vi "App - analyze RUS V6.vi"() -> ()   [LabVIEW 2021] (continued)
/LSCO22__130814c/5_Cooling_2nd_try/September_2014/091814/14.38000K_500_2500_2.10000V_0.00000T_Sep18-2014__05-14-56_001_091814.bin", "last mod"=timestamp(3493876496 s since 1904-01-01), "file name str"="D:\\Data\\Ultrasound\\LSCO\\LSCO22__130814c\\5_Cooling_2nd_try\\September_2014\\091814\\14.38000K_500_2500_2.10000V_0.00000T_Sep18-2014__05-14-56_001_091814.bin", "mod time(min)"=58231274.93333333, "file format"=enum."binary", "power(V)"=2.1, "Magn Field(T) "=0.0}, {"temperature"=14.384, "temperature str"="14.38400", "file path"=path "D:/Data/Ultrasound/LSCO/LSCO22__130814c/5_Cooling_2nd_try/September_2014/091814/14.38400K_500_2500_2.10000V_0.00000T_Sep18-2014__05-16-16_001_091814.bin", "last mod"=timestamp(3493876576 s since 1904-01-01), "file name str"="D:\\Data\\Ultrasound\\LSCO\\LSCO22__130814c\\5_Cooling_2nd_try\\September_2014\\091814\\14.38400K_500_2500_2.10000V_0.00000T_Sep18-2014__05-16-16_001_091814.bin", "mod time(min)"=58231276.266666666, "file format"=enum."binary", "power(V)"=2.1, "Magn Field(T) "=0.0}, {"temperature"=14.382, "temperature str"="14.38200", "file path"=path "D:/Data/Ultrasound/LSCO/LSCO22__130814c/5_Cooling_2nd_try/September_2014/091814/14.38200K_500_2500_2.10000V_0.00000T_Sep18-2014__05-17-35_001_091814.bin", "last mod"=timestamp(3493876655 s since 1904-01-01), "file name str"="D:\\Data\\Ultrasound\\LSCO\\LSCO22__130814c\\5_Cooling_2nd_try\\September_2014\\091814\\14.38200K_500_2500_2.10000V_0.00000T_Sep18-2014__05-17-35_001_091814.bin", "mod time(min)"=58231277.583333336, "file format"=enum."binary", "power(V)"=2.1, "Magn Field(T) "=0.0}, {"temperature"=14.383, "temperature str"="14.38300", "file path"=path "D:/Data/Ultrasound/LSCO/LSCO22__130814c/5_Cooling_2nd_try/September_2014/091814/14.38300K_500_2500_2.10000V_0.00000T_Sep18-2014__05-18-54_001_091814.bin", "last mod"=timestamp(3493876734 s since 1904-01-01), "file name str"="D:\\Data\\Ultrasound\\LSCO\\LSCO22__130814c\\5_Cooling_2nd_try\\September_2014\\091814\\14.38300K_500_2500_2.10000V_0.00000T_Sep18-2014__05-18-54_001_091814.bin", "mod time(min)"=58231278.9, "file format"=enum."binary", "power(V)"=2.1, "Magn Field(T) "=0.0}, {"temperature"=14.382, "temperature str"="14.38200", "file path"=path "D:/Data/Ultrasound/LSCO/LSCO22__130814c/5_Cooling_2nd_try/September_2014/091814/14.38200K_500_2500_2.10000V_0.00000T_Sep18-2014__05-20-14_001_091814.bin", "last mod"=timestamp(3493876814 s since 1904-01-01), "file name str"="D:\\Data\\Ultrasound\\LSCO\\LSCO22__130814c\\5_Cooling_2nd_try\\September_2014\\091814\\14.38200K_500_2500_2.10000V_0.00000T_Sep18-2014__05-20-14_001_091814.bin", "mod time(min)"=58231280.233333334, "file format"=enum."binary", "power(V)"=2.1, "Magn Field(T) "=0.0}, {"temperature"=14.381, "temperature str"="14.38100", "file path"=path "D:/Data/Ultrasound/LSCO/LSCO22__130814c/5_Cooling_2nd_try/September_2014/091814/14.38100K_500_2500_2.10000V_0.00000T_Sep18-2014__05-21-33_001_091814.bin", "last mod"=timestamp(3493876893 s since 1904-01-01), "file name str"="D:\\Data\\Ultrasound\\LSCO\\LSCO22__130814c\\5_Cooling_2nd_try\\September_2014\\091814\\14.38100K_500_2500_2.10000V_0.00000T_Sep18-2014__05-21-33_001_091814.bin", "mod time(min)"=58231281.55, "file format"=enum."binary", "power(V)"=2.1, "Magn Field(T) "=0.0}, {"temperature"=14.386, "temperature str"="14.38600", "file path"=path "D:/Data/Ultrasound/LSCO/LSCO22__130814c/5_Cooling_2nd_try/September_2014/091814/14.38600K_500_2500_2.10000V_0.00000T_Sep18-2014__05-22-52_001_091814.bin", "last mod"=timestamp(3493876972 s since 1904-01-01), "file name str"="D:\\Data\\Ultrasound\\LSCO\\LSCO22__130814c\\5_Cooling_2nd_try\\September_2014\\091814\\14.38600K_500_2500_2.10000V_0.00000T_Sep18-2014__05-22-52_001_091814.bin", "mod time(min)"=58231282.86666667, "file format"=enum."binary", "power(V)"=2.1, "Magn Field(T) "=0.0}, {"temperature"=14.389, "temperature str"="14.38900", "file path"=path "D:/Data/Ultrasound/LSCO/LSCO22__130814c/5_Cooling_2nd_try/September_2014/091814/14.38900K_500_2500_2.10000V_0.00000T_Sep18-2014__05-24-12_001_091814.bin", "last mod"=timestamp(3493877052 s since 1904-01-01), "file name str"="D:\\Data\\Ultrasound\\LSCO\\LSCO22__130814c\\5_Cooling_2nd_try\\September_2014\\091814\\14.38900K_500_2500_2.10000V_0.00000T_Sep18-2014__05-24-12_001_091814.bin", "mod time(min)"=58231284.2, "file format"=enum."binary", "power(V)"=2.1, "Magn Field(T) "=0.0}, {"temperature"=14.392, "temperature str"="14.39200", "file path"=path "D:/Data/Ultrasound/LSCO/LSCO22__130814c/5_Cooling_2nd_try/September_2014/091814/14.39200K_500_2500_2.10000V_0.00000T_Sep18-2014__05-25-31_001_091814.bin", "last mod"=timestamp(3493877131 s since 1904-01-01), "file name str"="D:\\Data\\Ultrasound\\LSCO\\LSCO22__130814c\\5_Cooling_2nd_try\\September_2014\\091814\\14.39200K_500_2500_2.10000V_0.00000T_Sep18-2014__05-25-31_001_091814.bin", "mod time(min)"=58231285.516666666, "file format"=enum."binary", "power(V)"=2.1, "Magn Field(T) "=0.0}, {"temperature"=14.395, "temperature str"="14.39500", "file path"=path "D:/Data/Ultrasound/LSCO/LSCO22__130814c/5_Cooling_2nd_try/September_2014/091814/14.39500K_500_2500_2.10000V_0.00000T_Sep18-2014__05-26-51_001_091814.bin", "last mod"=timestamp(3493877211 s since 1904-01-01), "file name str"="D:\\Data\\Ultrasound\\LSCO\\LSCO22__130814c\\5_Cooling_2nd_try\\September_2014\\091814\\14.39500K_500_2500_2.10000V_0.00000T_Sep18-2014__05-26-51_001_091814.bin", "mod time(min)"=58231286.85, "file format"=enum."binary", "power(V)"=2.1, "Magn Field(T) "=0.0}, {"temperature"=14.397, "temperature str"="14.39700", "file path"=path "D:/Data/Ultrasound/LSCO/LSCO22__130814c/5_Cooling_2nd_try/September_2014/091814/14.39700K_500_2500_2.10000V_0.00000T_Sep18-2014__05-28-10_001_091814.bin", "last mod"=timestamp(3493877290 s since 1904-01-01), "file name str"="D:\\Data\\Ultrasound\\LSCO\\LSCO22__130814c\\5_Cooling_2nd_try\\September_2014\\091814\\14.39700K_500_2500_2.10000V_0.00000T_Sep18-2014__05-28-10_001_091814.bin", "mod time(min)"=58231288.166666664, "file format"=enum."binary", "power(V)"=2.1, "Magn Field(T) "=0.0}, {"temperature"=14.399, "temperature str"="14.39900", "file path"=path "D:/Data/Ultrasound/LSCO/LSCO22__130814c/5_Cooling_2nd_try/September_2014/091814/14.39900K_500_2500_2.10000V_0.00000T_Sep18-2014__05-29-29_001_091814.bin", "last mod"=timestamp(3493877369 s since 1904-01-01), "file name str"="D:\\Data\\Ultrasound\\LSCO\\LSCO22__130814c\\5_Cooling_2nd_try\\September_2014\\091814\\14.39900K_500_2500_2.10000V_0.00000T_Sep18-2014__05-29-29_001_091814.bin", "mod time(min)"=58231289.483333334, "file format"=enum."binary", "power(V)"=2.1, "Magn Field(T) "=0.0}, {"temperature"=14.4, "temperature str"="14.40000", "file path"=path "D:/Data/Ultrasound/LSCO/LSCO22__130814c/5_Cooling_2nd_try/September_2014/091814/14.40000K_500_2500_2.10000V_0.00000T_Sep18-2014__05-30-49_001_091814.bin", "last mod"=timestamp(3493877449 s since 1904-01-01), "file name str"="D:\\Data\\Ultrasound\\LSCO\\LSCO22__130814c\\5_Cooling_2nd_try\\September_2014\\091814\\14.40000K_500_2500_2.10000V_0.00000T_Sep18-2014__05-30-49_001_091814.bin", "mod time(min)"=58231290.81666667, "file format"=enum."binary", "power(V)"=2.1, "Magn Field(T) "=0.0}, {"temperature"=14.404, "temperature str"="14.40400", "file path"=path "D:/Data/Ultrasound/LSCO/LSCO22__130814c/5_Cooling_2nd_try/September_2014/091814/14.40400K_500_2500_2.10000V_0.00000T_Sep18-2014__05-32-08_001_091814.bin", "last mod"=timestamp(3493877528 s since 1904-01-01), "file name str"="D:\\Data\\Ultrasound\\LSCO\\LSCO22__130814c\\5_Cooling_2nd_try\\September_2014\\091814\\14.40400K_500_2500_2.10000V_0.00000T_Sep18-2014__05-32-08_001_091814.bin", "mod time(min)"=58231292.13333333, "file format"=enum."binary", "power(V)"=2.1, "Magn Field(T) "=0.0}, {"temperature"=14.405, "temperature str"="14.40500", "file path"=path "D:/Data/Ultrasound/LSCO/LSCO22__130814c/5_Cooling_2nd_try/September_2014/091814/14.40500K_500_2500_2.10000V_0.00000T_Sep18-2014__05-33-28_001_091814.bin", "last mod"=timestamp(3493877608 s since 1904-01-01), "file name str"="D:\\Data\\Ultrasound\\LSCO\\LSCO22__130814c\\5_Cooling_2nd_try\\September_2014\\091814\\14.40500K_500_2500_2.10000V_0.00000T_Sep18-2014__05-33-28_001_091814.bin", "mod time(min)"=58231293.46666667, "file format"=enum."binary", "power(V)"=2.1, "Magn Field(T) "=0.0}, {"temperature"=14.407, "temperature str"="14.40700", "file path"=path "D:/Data/Ultrasound/LSCO/LSCO22__130814c/5_Cooling_2nd_try/September_2014/091814/14.40700K_500_2500_2.10000V_0.00000T_Sep18-2014__05-34-47_001_091814.bin", "last mod"=timestamp(3493877687 s since 1904-01-01), "file name str"="D:\\Data\\Ultrasound\\LSCO\\LSCO22__130814c\\5_Cooling_2nd_try\\September_2014\\091814\\14.40700K_500_2500_2.10000V_0.00000T_Sep18-2014__05-34-47_001_091814.bin", "mod time(min)"=58231294.78333333, "file format"=enum."binary", "power(V)"=2.1, "Magn Field(T) "=0.0}, {"temperature"=14.411, "temperature str"="14.41100", "file path"=path "D:/Data/Ultrasound/LSCO/LSCO22__130814c/5_Cooling_2nd_try/September_2014/091814/14.41100K_500_2500_2.10000V_0.00000T_Sep18-2014__05-36-06_001_091814.bin", "last mod"=timestamp(3493877766 s since 1904-01-01), "file name str"="D:\\Data\\Ultrasound\\LSCO\\LSCO22__130814c\\5_Cooling_2nd_try\\September_2014\\091814\\14.41100K_500_2500_2.10000V_0.00000T_Sep18-2014__05-36-06_001_091814.bin", "mod time(min)"=58231296.1, "file format"=enum."binary", "power(V)"=2.1, "Magn Field(T) "=0.0}, {"temperature"=14.416, "temperature str"="14.41600", "file path"=path "D:/Data/Ultrasound/LSCO/LSCO22__130814c/5_Cooling_2nd_try/September_2014/091814/14.41600K_500_2500_2.10000V_0.00000T_Sep18-2014__05-37-26_001_091814.bin", "last mod"=timestamp(3493877846 s since 1904-01-01), "file name str"="D:\\Data\\Ultrasound\\LSCO\\LSCO22__130814c\\5_Cooling_2nd_try\\September_2014\\091814\\14.41600K_500_2500_2.10000V_0.00000T_Sep18-2014__05-37-26_001_091814.bin", "mod time(min)"=58231297.43333333, "file format"=enum."binary", "power(V)"=2.1, "Magn Field(T) "=0.0}, {"temperature"=14.42, "temperature str"="14.42000", "file path"=path "D:/Data/Ultrasound/LSCO/LSCO22__130814c/5_Cooling_2nd_try/September_2014/091814/14.42000K_500_2500_2.10000V_0.00000T_Sep18-2014__05-38-45_001_091814.bin", "last mod"=timestamp(3493877925 s since 1904-01-01), "file name str"="D:\\Data\\Ultrasound\\LSCO\\LSCO22__130814c\\5_Cooling_2nd_try\\September_2014\\091814\\14.42000K_500_2500_2.10000V_0.00000T_Sep18-2014__05-38-45_001_091814.bin", "mod time(min)"=58231298.75, "file format"=enum."binary", "power(V)"=2.1, "Magn Field(T) "=0.0}, {"temperature"=14.42, "temperature str"="14.42000", "file path"=path "D:/Data/Ultrasound/LSCO/LSCO22__130814c/5_Cooling_2nd_try/September_2014/091814/14.42000K_500_2500_2.10000V_0.00000T_Sep18-2014__05-40-04_001_091814.bin", "last mod"=timestamp(3493878004 s since 1904-01-01), "file name str"="D:\\Data\\Ultrasound\\LSCO\\LSCO22__130814c\\5_Cooling_2nd_try\\September_2014\\091814\\14.42000K_500_2500_2.10000V_0.00000T_Sep18-2014__05-40-04_001_091814.bin", "mod time(min)"=58231300.06666667, "file format"=enum."binary", "power(V)"=2.1, "Magn Field(T) "=0.0}, {"temperature"=14.42, "temperature str"="14.42000", "file path"=path "D:/Data/Ultrasound/LSCO/LSCO22__130814c/5_Cooling_2nd_try/September_2014/091814/14.42000K_500_2500_2.10000V_0.00000T_Sep18-2014__05-41-24_001_091814.bin", "last mod"=timestamp(3493878084 s since 1904-01-01), "file name str"="D:\\Data\\Ultrasound\\LSCO\\LSCO22__130814c\\5_Cooling_2nd_try\\September_2014\\091814\\14.42000K_500_2500_2.10000V_0.00000T_Sep18-2014__05-41-24_001_091814.bin", "mod time(min)"=58231301.4, "file format"=enum."binary", "power(V)"=2.1, "Magn Field(T) "=0.0}, {"temperature"=14.42, "temperature str"="14.42000", "file path"=path "D:/Data/Ultrasound/LSCO/LSCO22__130814c/5_Cooling_2nd_try/September_2014/091814/14.42000K_500_2500_2.10000V_0.00000T_Sep18-2014__05-42-43_001_091814.bin", "last mod"=timestamp(3493878163 s since 1904-01-01), "file name str"="D:\\Data\\Ultrasound\\LSCO\\LSCO22__130814c\\5_Cooling_2nd_try\\September_2014\\091814\\14.42000K_500_2500_2.10000V_0.00000T_Sep18-2014__05-42-43_001_091814.bin", "mod time(min)"=58231302.71666667, "file format"=enum."binary", "power(V)"=2.1, "Magn Field(T) "=0.0}, {"temperature"=14.426, "temperature str"="14.42600", "file path"=path "D:/Data/Ultrasound/LSCO/LSCO22__130814c/5_Cooling_2nd_try/September_2014/091814/14.42600K_500_2500_2.10000V_0.00000T_Sep18-2014__05-44-03_001_091814.bin", "last mod"=timestamp(3493878243 s since 1904-01-01), "file name str"="D:\\Data\\Ultrasound\\LSCO\\LSCO22__130814c\\5_Cooling_2nd_try\\September_2014\\091814\\14.42600K_500_2500_2.10000V_0.00000T_Sep18-2014__05-44-03_001_091814.bin", "mod time(min)"=58231304.05, "file format"=enum."binary", "power(V)"=2.1, "Magn Field(T) "=0.0}, {"temperature"=14.427, "temperature str"="14.42700", "file path"=path "D:/Data/Ultrasound/LSCO/LSCO22__130814c/5_Cooling_2nd_try/September_2014/091814/14.42700K_500_2500_2.10000V_0.00000T_Sep18-2014__05-45-22_001_091814.bin", "last mod"=timestamp(3493878322 s since 1904-01-01), "file name str"="D:\\Data\\Ultrasound\\LSCO\\LSCO22__130814c\\5_Cooling_2nd_try\\September_2014\\091814\\14.42700K_500_2500_2.10000V_0.00000T_Sep18-2014__05-45-22_001_091814.bin", "mod time(min)"=58231305.36666667, "file format"=enum."binary", "power(V)"=2.1, "Magn Field(T) "=0.0}, {"temperature"=14.431, "temperature str"="14.43100", "file path"=path "D:/Data/Ultrasound/LSCO/LSCO22__130814c/5_Cooling_2nd_try/September_2014/091814/14.43100K_500_2500_2.10000V_0.00000T_Sep18-2014__05-46-41_001_091814.bin", "last mod"=timestamp(3493878401 s since 1904-01-01), "file name str"="D:\\Data\\Ultrasound\\LSCO\\LSCO22__130814c\\5_Cooling_2nd_try\\September_2014\\091814\\14.43100K_500_2500_2.10000V_0.00000T_Sep18-2014__05-46-41_001_091814.bin", "mod time(min)"=58231306.68333333, "file format"=enum."binary", "power(V)"=2.1, "Magn Field(T) "=0.0}, {"temperature"=14.43, "temperature str"="14.43000", "file path"=path "D:/Data/Ultrasound/LSCO/LSCO22__130814c/5_Cooling_2nd_try/September_2014/091814/14.43000K_500_2500_2.10000V_0.00000T_Sep18-2014__05-48-01_001_091814.bin", "last mod"=timestamp(3493878481 s since 1904-01-01), "file name str"="D:\\Data\\Ultrasound\\LSCO\\LSCO22__130814c\\5_Cooling_2nd_try\\September_2014\\091814\\14.43000K_500_2500_2.10000V_0.00000T_Sep18-2014__05-48-01_001_091814.bin", "mod time(min)"=58231308.016666666, "file format"=enum."binary", "power(V)"=2.1, "Magn Field(T) "=0.0}, {"temperature"=14.431, "temperature str"="14.43100", "file path"=path "D:/Data/Ultrasound/LSCO/LSCO22__130814c/5_Cooling_2nd_try/September_2014/091814/14.43100K_500_2500_2.10000V_0.00000T_Sep18-2014__05-49-20_001_091814.bin", "last mod"=timestamp(3493878560 s since 1904-01-01), "file name str"="D:\\Data\\Ultrasound\\LSCO\\LSCO22__130814c\\5_Cooling_2nd_try\\September_2014\\091814\\14.43100K_500_2500_2.10000V_0.00000T_Sep18-2014__05-49-20_001_091814.bin", "mod time(min)"=58231309.333333336, "file format"=enum."binary", "power(V)"=2.1, "Magn Field(T) "=0.0}, {"temperature"=14.433, "temperature str"="14.43300", "file path"=path "D:/Data/Ultrasound/LSCO/LSCO22__130814c/5_Cooling_2nd_try/September_2014/091814/14.43300K_500_2500_2.10000V_0.00000T_Sep18-2014__05-50-40_001_091814.bin", "last mod"=timestamp(3493878640 s since 1904-01-01), "file name str"="D:\\Data\\Ultrasound\\LSCO\\LSCO22__130814c\\5_Cooling_2nd_try\\September_2014\\091814\\14.43300K_500_2500_2.10000V_0.00000T_Sep18-2014__05-50-40_001_091814.bin", "mod time(min)"=58231310.666666664, "file format"=enum."binary", "power(V)"=2.1, "Magn Field(T) "=0.0}, {"temperature"=14.438, "temperature str"="14.43800", "file path"=path "D:/Data/Ultrasound/LSCO/LSCO22__130814c/5_Cooling_2nd_try/September_2014/091814/14.43800K_500_2500_2.10000V_0.00000T_Sep18-2014__05-51-59_001_091814.bin", "last mod"=timestamp(3493878719 s since 1904-01-01), "file name str"="D:\\Data\\Ultrasound\\LSCO\\LSCO22__130814c\\5_Cooling_2nd_try\\September_2014\\091814\\14.43800K_500_2500_2.10000V_0.00000T_Sep18-2014__05-51-59_001_091814.bin", "mod time(min)"=58231311.983333334, "file format"=enum."binary", "power(V)"=2.1, "Magn Field(T) "=0.0}, {"temperature"=14.434, "temperature str"="14.43400", "file path"=path "D:/Data/Ultrasound/LSCO/LSCO22__130814c/5_Cooling_2nd_try/September_2014/091814/14.43400K_500_2500_2.10000V_0.00000T_Sep18-2014__05-53-18_001_091814.bin", "last mod"=timestamp(3493878798 s since 1904-01-01), "file name str"="D:\\Data\\Ultrasound\\LSCO\\LSCO22__130814c\\5_Cooling_2nd_try\\September_2014\\091814\\14.43400K_500_2500_2.10000V_0.00000T_Sep18-2014__05-53-18_001_091814.bin", "mod time(min)"=58231313.3, "file format"=enum."binary", "power(V)"=2.1, "Magn Field(T) "=0.0}, {"temperature"=14.438, "temperature str"="14.43800", "file path"=path "D:/Data/Ultrasound/LSCO/LSCO22__130814c/5_Cooling_2nd_try/September_2014/091814/14.43800K_500_2500_2.10000V_0.00000T_Sep18-2014__05-54-38_001_091814.bin", "last mod"=timestamp(3493878878 s since 1904-01-01), "file name str"="D:\\Data\\Ultrasound\\LSCO\\LSCO22__130814c\\5_Cooling_2nd_try\\September_2014\\091814\\14.43800K_500_2500_2.10000V_0.00000T_Sep18-2014__05-54-38_001_091814.bin", "mod time(min)"=58231314.63333333, "file format"=enum."binary", "power(V)"=2.1, "Magn Field(T) "=0.0}, {"temperature"=14.441, "temperature str"="14.44100", "file path"=path "D:/Data/Ultrasound/LSCO/LSCO22__130814c/5_Cooling_2nd_try/September_2014/091814/14.44100K_500_2500_2.10000V_0.00000T_Sep18-2014__05-55-57_001_091814.bin", "last mod"=timestamp(3493878957 s since 1904-01-01), "file name str"="D:\\Data\\Ultrasound\\LSCO\\LSCO22__130814c\\5_Cooling_2nd_try\\September_2014\\091814\\14.44100K_500_2500_2.10000V_0.00000T_Sep18-2014__05-55-57_001_091814.bin", "mod time(min)"=58231315.95, "file format"=enum."binary", "power(V)"=2.1, "Magn Field(T) "=0.0}, {"temperature"=14.441, "temperature str"="14.44100", "file path"=path "D:/Data/Ultrasound/LSCO/LSCO22__130814c/5_Cooling_2nd_try/September_2014/091814/14.44100K_500_2500_2.10000V_0.00000T_Sep18-2014__05-57-16_001_091814.bin", "last mod"=timestamp(3493879036 s since 1904-01-01), "file name str"="D:\\Data\\Ultrasound\\LSCO\\LSCO22__130814c\\5_Cooling_2nd_try\\September_2014\\091814\\14.44100K_500_2500_2.10000V_0.00000T_Sep18-2014__05-57-16_001_091814.bin", "mod time(min)"=58231317.266666666, "file format"=enum."binary", "power(V)"=2.1, "Magn Field(T) "=0.0}, {"temperature"=14.444, "temperature str"="14.44400", "file path"=path "D:/Data/Ultrasound/LSCO/LSCO22__130814c/5_Cooling_2nd_try/September_2014/091814/14.44400K_500_2500_2.10000V_0.00000T_Sep18-2014__05-58-36_001_091814.bin", "last mod"=timestamp(3493879116 s since 1904-01-01), "file name str"="D:\\Data\\Ultrasound\\LSCO\\LSCO22__130814c\\5_Cooling_2nd_try\\September_2014\\091814\\14.44400K_500_2500_2.10000V_0.00000T_Sep18-2014__05-58-36_001_091814.bin", "mod time(min)"=58231318.6, "file format"=enum."binary", "power(V)"=2.1, "Magn Field(T) "=0.0}, {"temperature"=14.44, "temperature str"="14.44000", "file path"=path "D:/Data/Ultrasound/LSCO/LSCO22__130814c/5_Cooling_2nd_try/September_2014/091814/14.44000K_500_2500_2.10000V_0.00000T_Sep18-2014__05-59-55_001_091814.bin", "last mod"=timestamp(3493879195 s since 1904-01-01), "file name str"="D:\\Data\\Ultrasound\\LSCO\\LSCO22__130814c\\5_Cooling_2nd_try\\September_2014\\091814\\14.44000K_500_2500_2.10000V_0.00000T_Sep18-2014__05-59-55_001_091814.bin", "mod time(min)"=58231319.916666664, "file format"=enum."binary", "power(V)"=2.1, "Magn Field(T) "=0.0}, {"temperature"=14.446, "temperature str"="14.44600", "file path"=path "D:/Data/Ultrasound/LSCO/LSCO22__130814c/5_Cooling_2nd_try/September_2014/091814/14.44600K_500_2500_2.10000V_0.00000T_Sep18-2014__06-01-15_001_091814.bin", "last mod"=timestamp(3493879275 s since 1904-01-01), "file name str"="D:\\Data\\Ultrasound\\LSCO\\LSCO22__130814c\\5_Cooling_2nd_try\\September_2014\\091814\\14.44600K_500_2500_2.10000V_0.00000T_Sep18-2014__06-01-15_001_091814.bin", "mod time(min)"=58231321.25, "file format"=enum."binary", "power(V)"=2.1, "Magn Field(T) "=0.0}, {"temperature"=14.449, "temperature str"="14.44900", "file path"=path "D:/Data/Ultrasound/LSCO/LSCO22__130814c/5_Cooling_2nd_try/September_2014/091814/14.44900K_500_2500_2.10000V_0.00000T_Sep18-2014__06-02-34_001_091814.bin", "last mod"=timestamp(3493879354 s since 1904-01-01), "file name str"="D:\\Data\\Ultrasound\\LSCO\\LSCO22__130814c\\5_Cooling_2nd_try\\September_2014\\091814\\14.44900K_500_2500_2.10000V_0.00000T_Sep18-2014__06-02-34_001_091814.bin", "mod time(min)"=58231322.56666667, "file format"=enum."binary", "power(V)"=2.1, "Magn Field(T) "=0.0}, {"temperature"=14.447, "temperature str"="14.44700", "file path"=path "D:/Data/Ultrasound/LSCO/LSCO22__130814c/5_Cooling_2nd_try/September_2014/091814/14.44700K_500_2500_2.10000V_0.00000T_Sep18-2014__06-03-53_001_091814.bin", "last mod"=timestamp(3493879433 s since 1904-01-01), "file name str"="D:\\Data\\Ultrasound\\LSCO\\LSCO22__130814c\\5_Cooling_2nd_try\\September_2014\\091814\\14.44700K_500_2500_2.10000V_0.00000T_Sep18-2014__06-03-53_001_091814.bin", "mod time(min)"=58231323.88333333, "file format"=enum."binary", "power(V)"=2.1, "Magn Field(T) "=0.0}, {"temperature"=14.448, "temperature str"="14.44800", "file path"=path "D:/Data/Ultrasound/LSCO/LSCO22__130814c/5_Cooling_2nd_try/September_2014/091814/14.44800K_500_2500_2.10000V_0.00000T_Sep18-2014__06-05-13_001_091814.bin", "last mod"=timestamp(3493879513 s since 1904-01-01), "file name str"="D:\\Data\\Ultrasound\\LSCO\\LSCO22__130814c\\5_Cooling_2nd_try\\September_2014\\091814\\14.44800K_500_2500_2.10000V_0.00000T_Sep18-2014__06-05-13_001_091814.bin", "mod time(min)"=58231325.21666667, "file format"=enum."binary", "power(V)"=2.1, "Magn Field(T) "=0.0}, {"temperature"=14.453, "temperature str"="14.45300", "file path"=path "D:/Data/Ultrasound/LSCO/LSCO22__130814c/5_Cooling_2nd_try/September_2014/091814/14.45300K_500_2500_2.10000V_0.00000T_Sep18-2014__06-06-32_001_091814.bin", "last mod"=timestamp(3493879592 s since 1904-01-01), "file name str"="D:\\Data\\Ultrasound\\LSCO\\LSCO22__130814c\\5_Cooling_2nd_try\\September_2014\\091814\\14.45300K_500_2500_2.10000V_0.00000T_Sep18-2014__06-06-32_001_091814.bin", "mod time(min)"=58231326.53333333, "file format"=enum."binary", "power(V)"=2.1, "Magn Field(T) "=0.0}, {"temperature"=14.45, "temperature str"="14.45000", "file path"=path "D:/Data/Ultrasound/LSCO/LSCO22__130814c/5_Cooling_2nd_try/September_2014/091814/14.45000K_500_2500_2.10000V_0.00000T_Sep18-2014__06-07-51_001_091814.bin", "last mod"=timestamp(3493879671 s since 1904-01-01), "file name str"="D:\\Data\\Ultrasound\\LSCO\\LSCO22__130814c\\5_Cooling_2nd_try\\September_2014\\091814\\14.45000K_500_2500_2.10000V_0.00000T_Sep18-2014__06-07-51_001_091814.bin", "mod time(min)"=58231327.85, "file format"=enum."binary", "power(V)"=2.1, "Magn Field(T) "=0.0}, {"temperature"=14.451, "temperature str"="14.45100", "file path"=path "D:/Data/Ultrasound/LSCO/LSCO22__130814c/5_Cooling_2nd_try/September_2014/091814/14.45100K_500_2500_2.10000V_0.00000T_Sep18-2014__06-09-11_001_091814.bin", "last mod"=timestamp(3493879751 s since 1904-01-01), "file name str"="D:\\Data\\Ultrasound\\LSCO\\LSCO22__130814c\\5_Cooling_2nd_try\\September_2014\\091814\\14.45100K_500_2500_2.10000V_0.00000T_Sep18-2014__06-09-11_001_091814.bin", "mod time(min)"=58231329.18333333, "file format"=enum."binary", "power(V)"=2.1, "Magn Field(T) "=0.0}, {"temperature"=14.449, "temperature str"="14.44900", "file path"=path "D:/Data/Ultrasound/LSCO/LSCO22__130814c/5_Cooling_2nd_try/September_2014/091814/14.44900K_500_2500_2.10000V_0.00000T_Sep18-2014__06-10-30_001_091814.bin", "last mod"=timestamp(3493879830 s since 1904-01-01), "file name str"="D:\\Data\\Ultrasound\\LSCO\\LSCO22__130814c\\5_Cooling_2nd_try\\September_2014\\091814\\14.44900K_500_2500_2.10000V_0.00000T_Sep18-2014__06-10-30_001_091814.bin", "mod time(min)"=58231330.5, "file format"=enum."binary", "power(V)"=2.1, "Magn Field(T) "=0.0}, {"temperature"=14.45, "temperature str"="14.45000", "file path"=path "D:/Data/Ultrasound/LSCO/LSCO22__130814c/5_Cooling_2nd_try/September_2014/091814/14.45000K_500_2500_2.10000V_0.00000T_Sep18-2014__06-11-50_001_091814.bin", "last mod"=timestamp(3493879910 s since 1904-01-01), "file name str"="D:\\Data\\Ultrasound\\LSCO\\LSCO22__130814c\\5_Cooling_2nd_try\\September_2014\\091814\\14.45000K_500_2500_2.10000V_0.00000T_Sep18-2014__06-11-50_001_091814.bin", "mod time(min)"=58231331.833333336, "file format"=enum."binary", "power(V)"=2.1, "Magn Field(T) "=0.0}, {"temperature"=14.453, "temperature str"="14.45300", "file path"=path "D:/Data/Ultrasound/LSCO/LSCO22__130814c/5_Cooling_2nd_try/September_2014/091814/14.45300K_500_2500_2.10000V_0.00000T_Sep18-2014__06-13-09_001_091814.bin", "last mod"=timestamp(3493879989 s since 1904-01-01), "file name str"="D:\\Data\\Ultrasound\\LSCO\\LSCO22__130814c\\5_Cooling_2nd_try\\September_2014\\091814\\14.45300K_500_2500_2.10000V_0.00000T_Sep18-2014__06-13-09_001_091814.bin", "mod time(min)"=58231333.15, "file format"=enum."binary", "power(V)"=2.1, "Magn Field(T) "=0.0}, {"temperature"=14.455, "temperature str"="14.45500", "file path"=path "D:/Data/Ultrasound/LSCO/LSCO22__130814c/5_Cooling_2nd_try/September_2014/091814/14.45500K_500_2500_2.10000V_0.00000T_Sep18-2014__06-14-28_001_091814.bin", "last mod"=timestamp(3493880068 s since 1904-01-01), "file name str"="D:\\Data\\Ultrasound\\LSCO\\LSCO22__130814c\\5_Cooling_2nd_try\\September_2014\\091814\\14.45500K_500_2500_2.10000V_0.00000T_Sep18-2014__06-14-28_001_091814.bin", "mod time(min)"=58231334.46666667, "file format"=enum."binary", "power(V)"=2.1, "Magn Field(T) "=0.0}, {"temperature"=14.456, "temperature str"="14.45600", "file path"=path "D:/Data/Ultrasound/LSCO/LSCO22__130814c/5_Cooling_2nd_try/September_2014/091814/14.45600K_500_2500_2.10000V_0.00000T_Sep18-2014__06-15-48_001_091814.bin", "last mod"=timestamp(3493880148 s since 1904-01-01), "file name str"="D:\\Data\\Ultrasound\\LSCO\\LSCO22__130814c\\5_Cooling_2nd_try\\September_2014\\091814\\14.45600K_500_2500_2.10000V_0.00000T_Sep18-2014__06-15-48_001_091814.bin", "mod time(min)"=58231335.8, "file format"=enum."binary", "power(V)"=2.1, "Magn Field(T) "=0.0}, {"temperature"=14.457, "temperature str"="14.45700", "file path"=path "D:/Data/Ultrasound/LSCO/LSCO22__130814c/5_Cooling_2nd_try/September_2014/091814/14.45700K_500_2500_2.10000V_0.00000T_Sep18-2014__06-17-07_001_091814.bin", "last mod"=timestamp(3493880227 s since 1904-01-01), "file name str"="D:\\Data\\Ultrasound\\LSCO\\LSCO22__130814c\\5_Cooling_2nd_try\\September_2014\\091814\\14.45700K_500_2500_2.10000V_0.00000T_Sep18-2014__06-17-07_001_091814.bin", "mod time(min)"=58231337.11666667, "file format"=enum."binary", "power(V)"=2.1, "Magn Field(T) "=0.0}, {"temperature"=14.458, "temperature str"="14.45800", "file path"=path "D:/Data/Ultrasound/LSCO/LSCO22__130814c/5_Cooling_2nd_try/September_2014/091814/14.45800K_500_2500_2.10000V_0.00000T_Sep18-2014__06-18-27_001_091814.bin", "last mod"=timestamp(3493880307 s since 1904-01-01), "file name str"="D:\\Data\\Ultrasound\\LSCO\\LSCO22__130814c\\5_Cooling_2nd_try\\September_2014\\091814\\14.45800K_500_2500_2.10000V_0.00000T_Sep18-2014__06-18-27_001_091814.bin", "mod time(min)"=58231338.45, "file format"=enum."binary", "power(V)"=2.1, "Magn Field(T) "=0.0}, {"temperature"=14.455, "temperature str"="14.45500", "file path"=path "D:/Data/Ultrasound/LSCO/LSCO22__130814c/5_Cooling_2nd_try/September_2014/091814/14.45500K_500_2500_2.10000V_0.00000T_Sep18-2014__06-19-46_001_091814.bin", "last mod"=timestamp(3493880386 s since 1904-01-01), "file name str"="D:\\Data\\Ultrasound\\LSCO\\LSCO22__130814c\\5_Cooling_2nd_try\\September_2014\\091814\\14.45500K_500_2500_2.10000V_0.00000T_Sep18-2014__06-19-46_001_091814.bin", "mod time(min)"=58231339.766666666, "file format"=enum."binary", "power(V)"=2.1, "Magn Field(T) "=0.0}, {"temperature"=14.459, "temperature str"="14.45900", "file path"=path "D:/Data/Ultrasound/LSCO/LSCO22__130814c/5_Cooling_2nd_try/September_2014/091814/14.45900K_500_2500_2.10000V_0.00000T_Sep18-2014__06-21-05_001_091814.bin", "last mod"=timestamp(3493880465 s since 1904-01-01), "file name str"="D:\\Data\\Ultrasound\\LSCO\\LSCO22__130814c\\5_Cooling_2nd_try\\September_2014\\091814\\14.45900K_500_2500_2.10000V_0.00000T_Sep18-2014__06-21-05_001_091814.bin", "mod time(min)"=58231341.083333336, "file format"=enum."binary", "power(V)"=2.1, "Magn Field(T) "=0.0}, {"temperature"=14.46, "temperature str"="14.46000", "file path"=path "D:/Data/Ultrasound/LSCO/LSCO22__130814c/5_Cooling_2nd_try/September_2014/091814/14.46000K_500_2500_2.10000V_0.00000T_Sep18-2014__06-22-25_001_091814.bin", "last mod"=timestamp(3493880545 s since 1904-01-01), "file name str"="D:\\Data\\Ultrasound\\LSCO\\LSCO22__130814c\\5_Cooling_2nd_try\\September_2014\\091814\\14.46000K_500_2500_2.10000V_0.00000T_Sep18-2014__06-22-25_001_091814.bin", "mod time(min)"=58231342.416666664, "file format"=enum."binary", "power(V)"=2.1, "Magn Field(T) "=0.0}, {"temperature"=14.459, "temperature str"="14.45900", "file path"=path "D:/Data/Ultrasound/LSCO/LSCO22__130814c/5_Cooling_2nd_try/September_2014/091814/14.45900K_500_2500_2.10000V_0.00000T_Sep18-2014__06-23-44_001_091814.bin", "last mod"=timestamp(3493880624 s since 1904-01-01), "file name str"="D:\\Data\\Ultrasound\\LSCO\\LSCO22__130814c\\5_Cooling_2nd_try\\September_2014\\091814\\14.45900K_500_2500_2.10000V_0.00000T_Sep18-2014__06-23-44_001_091814.bin", "mod time(min)"=58231343.733333334, "file format"=enum."binary", "power(V)"=2.1, "Magn Field(T) "=0.0}, {"temperature"=14.461, "temperature str"="14.46100", "file path"=path "D:/Data/Ultrasound/LSCO/LSCO22__130814c/5_Cooling_2nd_try/September_2014/091814/14.46100K_500_2500_2.10000V_0.00000T_Sep18-2014__06-25-03_001_091814.bin", "last mod"=timestamp(3493880703 s since 1904-01-01), "file name str"="D:\\Data\\Ultrasound\\LSCO\\LSCO22__130814c\\5_Cooling_2nd_try\\September_2014\\091814\\14.46100K_500_2500_2.10000V_0.00000T_Sep18-2014__06-25-03_001_091814.bin", "mod time(min)"=58231345.05, "file format"=enum."binary", "power(V)"=2.1, "Magn Field(T) "=0.0}, {"temperature"=14.465, "temperature str"="14.46500", "file path"=path "D:/Data/Ultrasound/LSCO/LSCO22__130814c/5_Cooling_2nd_try/September_2014/091814/14.46500K_500_2500_2.10000V_0.00000T_Sep18-2014__06-26-23_001_091814.bin", "last mod"=timestamp(3493880783 s since 1904-01-01), "file name str"="D:\\Data\\Ultrasound\\LSCO\\LSCO22__130814c\\5_Cooling_2nd_try\\September_2014\\091814\\14.46500K_500_2500_2.10000V_0.00000T_Sep18-2014__06-26-23_001_091814.bin", "mod time(min)"=58231346.38333333, "file format"=enum."binary", "power(V)"=2.1, "Magn Field(T) "=0.0}, {"temperature"=14.467, "temperature str"="14.46700", "file path"=path "D:/Data/Ultrasound/LSCO/LSCO22__130814c/5_Cooling_2nd_try/September_2014/091814/14.46700K_500_2500_2.10000V_0.00000T_Sep18-2014__06-27-42_001_091814.bin", "last mod"=timestamp(3493880862 s since 1904-01-01), "file name str"="D:\\Data\\Ultrasound\\LSCO\\LSCO22__130814c\\5_Cooling_2nd_try\\September_2014\\091814\\14.46700K_500_2500_2.10000V_0.00000T_Sep18-2014__06-27-42_001_091814.bin", "mod time(min)"=58231347.7, "file format"=enum."binary", "power(V)"=2.1, "Magn Field(T) "=0.0}, {"temperature"=14.467, "temperature str"="14.46700", "file path"=path "D:/Data/Ultrasound/LSCO/LSCO22__130814c/5_Cooling_2nd_try/September_2014/091814/14.46700K_500_2500_2.10000V_0.00000T_Sep18-2014__06-29-02_001_091814.bin", "last mod"=timestamp(3493880942 s since 1904-01-01), "file name str"="D:\\Data\\Ultrasound\\LSCO\\LSCO22__130814c\\5_Cooling_2nd_try\\September_2014\\091814\\14.46700K_500_2500_2.10000V_0.00000T_Sep18-2014__06-29-02_001_091814.bin", "mod time(min)"=58231349.03333333, "file format"=enum."binary", "power(V)"=2.1, "Magn Field(T) "=0.0}, {"temperature"=14.469, "temperature str"="14.46900", "file path"=path "D:/Data/Ultrasound/LSCO/LSCO22__130814c/5_Cooling_2nd_try/September_2014/091814/14.46900K_500_2500_2.10000V_0.00000T_Sep18-2014__06-30-21_001_091814.bin", "last mod"=timestamp(3493881021 s since 1904-01-01), "file name str"="D:\\Data\\Ultrasound\\LSCO\\LSCO22__130814c\\5_Cooling_2nd_try\\September_2014\\091814\\14.46900K_500_2500_2.10000V_0.00000T_Sep18-2014__06-30-21_001_091814.bin", "mod time(min)"=58231350.35, "file format"=enum."binary", "power(V)"=2.1, "Magn Field(T) "=0.0}, {"temperature"=14.467, "temperature str"="14.46700", "file path"=path "D:/Data/Ultrasound/LSCO/LSCO22__130814c/5_Cooling_2nd_try/September_2014/091814/14.46700K_500_2500_2.10000V_0.00000T_Sep18-2014__06-31-40_001_091814.bin", "last mod"=timestamp(3493881100 s since 1904-01-01), "file name str"="D:\\Data\\Ultrasound\\LSCO\\LSCO22__130814c\\5_Cooling_2nd_try\\September_2014\\091814\\14.46700K_500_2500_2.10000V_0.00000T_Sep18-2014__06-31-40_001_091814.bin", "mod time(min)"=58231351.666666664, "file format"=enum."binary", "power(V)"=2.1, "Magn Field(T) "=0.0}, {"temperature"=14.467, "temperature str"="14.46700", "file path"=path "D:/Data/Ultrasound/LSCO/LSCO22__130814c/5_Cooling_2nd_try/September_2014/091814/14.46700K_500_2500_2.10000V_0.00000T_Sep18-2014__06-33-00_001_091814.bin", "last mod"=timestamp(3493881180 s since 1904-01-01), "file name str"="D:\\Data\\Ultrasound\\LSCO\\LSCO22__130814c\\5_Cooling_2nd_try\\September_2014\\091814\\14.46700K_500_2500_2.10000V_0.00000T_Sep18-2014__06-33-00_001_091814.bin", "mod time(min)"=58231353.0, "file format"=enum."binary", "power(V)"=2.1, "Magn Field(T) "=0.0}, {"temperature"=14.469, "temperature str"="14.46900", "file path"=path "D:/Data/Ultrasound/LSCO/LSCO22__130814c/5_Cooling_2nd_try/September_2014/091814/14.46900K_500_2500_2.10000V_0.00000T_Sep18-2014__06-34-19_001_091814.bin", "last mod"=timestamp(3493881259 s since 1904-01-01), "file name str"="D:\\Data\\Ultrasound\\LSCO\\LSCO22__130814c\\5_Cooling_2nd_try\\September_2014\\091814\\14.46900K_500_2500_2.10000V_0.00000T_Sep18-2014__06-34-19_001_091814.bin", "mod time(min)"=58231354.31666667, "file format"=enum."binary", "power(V)"=2.1, "Magn Field(T) "=0.0}, {"temperature"=14.471, "temperature str"="14.47100", "file path"=path "D:/Data/Ultrasound/LSCO/LSCO22__130814c/5_Cooling_2nd_try/September_2014/091814/14.47100K_500_2500_2.10000V_0.00000T_Sep18-2014__06-35-39_001_091814.bin", "last mod"=timestamp(3493881339 s since 1904-01-01), "file name str"="D:\\Data\\Ultrasound\\LSCO\\LSCO22__130814c\\5_Cooling_2nd_try\\September_2014\\091814\\14.47100K_500_2500_2.10000V_0.00000T_Sep18-2014__06-35-39_001_091814.bin", "mod time(min)"=58231355.65, "file format"=enum."binary", "power(V)"=2.1, "Magn Field(T) "=0.0}, {"temperature"=14.473, "temperature str"="14.47300", "file path"=path "D:/Data/Ultrasound/LSCO/LSCO22__130814c/5_Cooling_2nd_try/September_2014/091814/14.47300K_500_2500_2.10000V_0.00000T_Sep18-2014__06-36-58_001_091814.bin", "last mod"=timestamp(3493881418 s since 1904-01-01), "file name str"="D:\\Data\\Ultrasound\\LSCO\\LSCO22__130814c\\5_Cooling_2nd_try\\September_2014\\091814\\14.47300K_500_2500_2.10000V_0.00000T_Sep18-2014__06-36-58_001_091814.bin", "mod time(min)"=58231356.96666667, "file format"=enum."binary", "power(V)"=2.1, "Magn Field(T) "=0.0}, {"temperature"=14.47, "temperature str"="14.47000", "file path"=path "D:/Data/Ultrasound/LSCO/LSCO22__130814c/5_Cooling_2nd_try/September_2014/091814/14.47000K_500_2500_2.10000V_0.00000T_Sep18-2014__06-38-17_001_091814.bin", "last mod"=timestamp(3493881497 s since 1904-01-01), "file name str"="D:\\Data\\Ultrasound\\LSCO\\LSCO22__130814c\\5_Cooling_2nd_try\\September_2014\\091814\\14.47000K_500_2500_2.10000V_0.00000T_Sep18-2014__06-38-17_001_091814.bin", "mod time(min)"=58231358.28333333, "file format"=enum."binary", "power(V)"=2.1, "Magn Field(T) "=0.0}, {"temperature"=14.474, "temperature str"="14.47400", "file path"=path "D:/Data/Ultrasound/LSCO/LSCO22__130814c/5_Cooling_2nd_try/September_2014/091814/14.47400K_500_2500_2.10000V_0.00000T_Sep18-2014__06-39-37_001_091814.bin", "last mod"=timestamp(3493881577 s since 1904-01-01), "file name str"="D:\\Data\\Ultrasound\\LSCO\\LSCO22__130814c\\5_Cooling_2nd_try\\September_2014\\091814\\14.47400K_500_2500_2.10000V_0.00000T_Sep18-2014__06-39-37_001_091814.bin", "mod time(min)"=58231359.61666667, "file format"=enum."binary", "power(V)"=2.1, "Magn Field(T) "=0.0}, {"temperature"=14.471, "temperature str"="14.47100", "file path"=path "D:/Data/Ultrasound/LSCO/LSCO22__130814c/5_Cooling_2nd_try/September_2014/091814/14.47100K_500_2500_2.10000V_0.00000T_Sep18-2014__06-40-56_001_091814.bin", "last mod"=timestamp(3493881656 s since 1904-01-01), "file name str"="D:\\Data\\Ultrasound\\LSCO\\LSCO22__130814c\\5_Cooling_2nd_try\\September_2014\\091814\\14.47100K_500_2500_2.10000V_0.00000T_Sep18-2014__06-40-56_001_091814.bin", "mod time(min)"=58231360.93333333, "file format"=enum."binary", "power(V)"=2.1, "Magn Field(T) "=0.0}, {"temperature"=14.471, "temperature str"="14.47100", "file path"=path "D:/Data/Ultrasound/LSCO/LSCO22__130814c/5_Cooling_2nd_try/September_2014/091814/14.47100K_500_2500_2.10000V_0.00000T_Sep18-2014__06-42-15_001_091814.bin", "last mod"=timestamp(3493881735 s since 1904-01-01), "file name str"="D:\\Data\\Ultrasound\\LSCO\\LSCO22__130814c\\5_Cooling_2nd_try\\September_2014\\091814\\14.47100K_500_2500_2.10000V_0.00000T_Sep18-2014__06-42-15_001_091814.bin", "mod time(min)"=58231362.25, "file format"=enum."binary", "power(V)"=2.1, "Magn Field(T) "=0.0}, {"temperature"=14.473, "temperature str"="14.47300", "file path"=path "D:/Data/Ultrasound/LSCO/LSCO22__130814c/5_Cooling_2nd_try/September_2014/091814/14.47300K_500_2500_2.10000V_0.00000T_Sep18-2014__06-43-35_001_091814.bin", "last mod"=timestamp(3493881815 s since 1904-01-01), "file name str"="D:\\Data\\Ultrasound\\LSCO\\LSCO22__130814c\\5_Cooling_2nd_try\\September_2014\\091814\\14.47300K_500_2500_2.10000V_0.00000T_Sep18-2014__06-43-35_001_091814.bin", "mod time(min)"=58231363.583333336, "file format"=enum."binary", "power(V)"=2.1, "Magn Field(T) "=0.0}, {"temperature"=14.476, "temperature str"="14.47600", "file path"=path "D:/Data/Ultrasound/LSCO/LSCO22__130814c/5_Cooling_2nd_try/September_2014/091814/14.47600K_500_2500_2.10000V_0.00000T_Sep18-2014__06-44-54_001_091814.bin", "last mod"=timestamp(3493881894 s since 1904-01-01), "file name str"="D:\\Data\\Ultrasound\\LSCO\\LSCO22__130814c\\5_Cooling_2nd_try\\September_2014\\091814\\14.47600K_500_2500_2.10000V_0.00000T_Sep18-2014__06-44-54_001_091814.bin", "mod time(min)"=58231364.9, "file format"=enum."binary", "power(V)"=2.1, "Magn Field(T) "=0.0}, {"temperature"=14.477, "temperature str"="14.47700", "file path"=path "D:/Data/Ultrasound/LSCO/LSCO22__130814c/5_Cooling_2nd_try/September_2014/091814/14.47700K_500_2500_2.10000V_0.00000T_Sep18-2014__06-46-14_001_091814.bin", "last mod"=timestamp(3493881974 s since 1904-01-01), "file name str"="D:\\Data\\Ultrasound\\LSCO\\LSCO22__130814c\\5_Cooling_2nd_try\\September_2014\\091814\\14.47700K_500_2500_2.10000V_0.00000T_Sep18-2014__06-46-14_001_091814.bin", "mod time(min)"=58231366.233333334, "file format"=enum."binary", "power(V)"=2.1, "Magn Field(T) "=0.0}, {"temperature"=14.479, "temperature str"="14.47900", "file path"=path "D:/Data/Ultrasound/LSCO/LSCO22__130814c/5_Cooling_2nd_try/September_2014/091814/14.47900K_500_2500_2.10000V_0.00000T_Sep18-2014__06-47-33_001_091814.bin", "last mod"=timestamp(3493882053 s since 1904-01-01), "file name str"="D:\\Data\\Ultrasound\\LSCO\\LSCO22__130814c\\5_Cooling_2nd_try\\September_2014\\091814\\14.47900K_500_2500_2.10000V_0.00000T_Sep18-2014__06-47-33_001_091814.bin", "mod time(min)"=58231367.55, "file format"=enum."binary", "power(V)"=2.1, "Magn Field(T) "=0.0}, {"temperature"=14.481, "temperature str"="14.48100", "file path"=path "D:/Data/Ultrasound/LSCO/LSCO22__130814c/5_Cooling_2nd_try/September_2014/091814/14.48100K_500_2500_2.10000V_0.00000T_Sep18-2014__06-48-52_001_091814.bin", "last mod"=timestamp(3493882132 s since 1904-01-01), "file name str"="D:\\Data\\Ultrasound\\LSCO\\LSCO22__130814c\\5_Cooling_2nd_try\\September_2014\\091814\\14.48100K_500_2500_2.10000V_0.00000T_Sep18-2014__06-48-52_001_091814.bin", 
